vi "Measure.vi"(8 "error in (no error)":errorcluster, 11 "QPS settings":T1={"TWM pipe name"="\\\\.\\pipe\\TWM:server", "Measurement properties"={"Measurement ID"=enum."1", "Description"="3 phase, 3 ADC, 1 PJVS", "Switching matrix M"=[], "Signal frequency  (Hz)"=50.0, "Signal amplitudes (V)"=[], "PRs"=1, "PRe"=10, "MRs"=0, "MRe"=0, "Set PJVS frequency (Hz)"=50.0, "PJVS reference voltages (1 period, V)"=[], "Requiested PJVS steps"=10, "Sampling f (Hz)"=7000.0}, "PJVS setup"={"PJVS type"=enum."AC-supraVOLTcontrol", "Status Refnum"=refnum, "Abort Refnum"=refnum, "AC-supraVOLTcontrol"={"IP address:port (0.0.0.0:0000)"="0.0.0.0:0000", "Timeouts"={"TCP Read & Write (ms)"=7000, "Sensors readout"=5000, "PJVS setup"=10000, "Nullmeter readout"=5000, "Multiplexer setup"=3000, "57XX setup"=15000, "Generator setup"=5000, "Synthesizer setup"=3000, "Sampler readout"=10000}, "Simulation mode"=FALSE, "Debug mode"=FALSE}, "NPL bias source"={"Server name"="CZC", "Bias setup file"=path ""}}} {"Measurement properties"."PJVS reference voltages (1 period, V)" format="%.9g"}) -> (0 "error out":errorcluster, 3 "QPS settings out":T1={"TWM pipe name"="\\\\.\\pipe\\TWM:server", "Measurement properties"={"Measurement ID"=enum."1", "Description"="3 phase, 3 ADC, 1 PJVS", "Switching matrix M"=[], "Signal frequency  (Hz)"=50.0, "Signal amplitudes (V)"=[], "PRs"=1, "PRe"=10, "MRs"=0, "MRe"=0, "Set PJVS frequency (Hz)"=50.0, "PJVS reference voltages (1 period, V)"=[], "Requiested PJVS steps"=10, "Sampling f (Hz)"=7000.0}, "PJVS setup"={"PJVS type"=enum."AC-supraVOLTcontrol", "Status Refnum"=refnum, "Abort Refnum"=refnum, "AC-supraVOLTcontrol"={"IP address:port (0.0.0.0:0000)"="0.0.0.0:0000", "Timeouts"={"TCP Read & Write (ms)"=7000, "Sensors readout"=5000, "PJVS setup"=10000, "Nullmeter readout"=5000, "Multiplexer setup"=3000, "57XX setup"=15000, "Generator setup"=5000, "Synthesizer setup"=3000, "Sampler readout"=10000}, "Simulation mode"=FALSE, "Debug mode"=FALSE}, "NPL bias source"={"Server name"="CZC", "Bias setup file"=path ""}}} {"Measurement properties"."PJVS reference voltages (1 period, V)" format="%.9g"})   [LabVIEW 2020]
uses:
  external libraries/TWM client.lvlibp
  Type definitions/Measurement ID.ctl
  Type definitions/Measuement properties.ctl
  General PJVS driver/Type definitions/PJVS Type.ctl
  PJVS drivers/acsvcontrol-driver/build/ACSVcontrol-driver_0.2.0.0.llb/Timeouts.ctl
  PJVS drivers/acsvcontrol-driver/build/ACSVcontrol-driver_0.2.0.0.llb/ACSVcontrol-driver.lvlib
  General PJVS driver/Type definitions/PJVS Setup.ctl
  General PJVS driver/QPSsettings.ctl
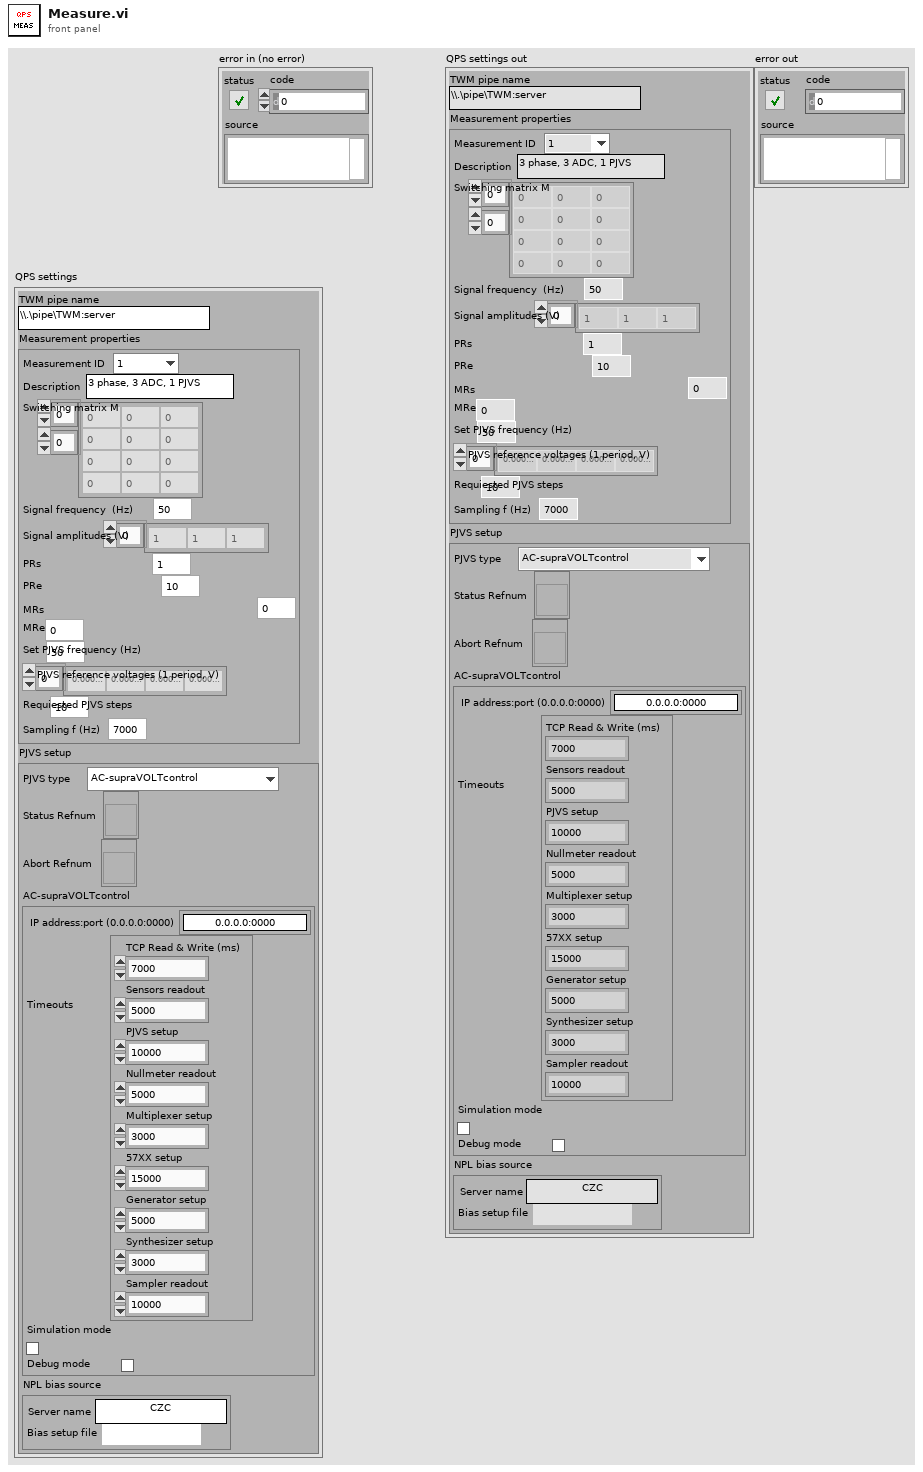
[diagram p1: front panel]
types:
  T1 = typedef "QPSsettings.ctl" = cluster{"TWM pipe name":string, "Measurement properties":T2, "PJVS setup":T4}
  T2 = typedef "Measuement properties.ctl" = cluster{"Measurement ID":T3, "Description":string, "Switching matrix M":i32[][], "Signal frequency  (Hz)":dbl, "Signal amplitudes (V)":dbl[], "PRs":i32, "PRe":i32, "MRs":i32, "MRe":i32, "Set PJVS frequency (Hz)":dbl, "PJVS reference voltages (1 period, V)":dbl[], "Requiested PJVS steps":i32, "Sampling f (Hz)":dbl}
  T3 = typedef "Measurement ID.ctl" = enum16{"M", "1", "2", "3"}
  T4 = typedef "PJVS Setup.ctl" = cluster{"PJVS type":T5, "Status Refnum":refnum<vi>, "Abort Refnum":refnum<vi>, "AC-supraVOLTcontrol":cluster{"IP address:port (0.0.0.0:0000)":string, "Timeouts":T6, "Simulation mode":bool, "Debug mode":bool}, "NPL bias source":cluster{"Server name":string, "Bias setup file":path}}
  T5 = typedef "PJVS Type.ctl" = enum16{"AC-supraVOLTcontrol", "NPL bias source"}
  T6 = typedef "ACSVcontrol-driver.lvlib/Timeouts.ctl" = cluster{"TCP Read & Write (ms)":i32, "Sensors readout":i32, "PJVS setup":i32, "Nullmeter readout":i32, "Multiplexer setup":i32, "57XX setup":i32, "Generator setup":i32, "Synthesizer setup":i32, "Sampler readout":i32}
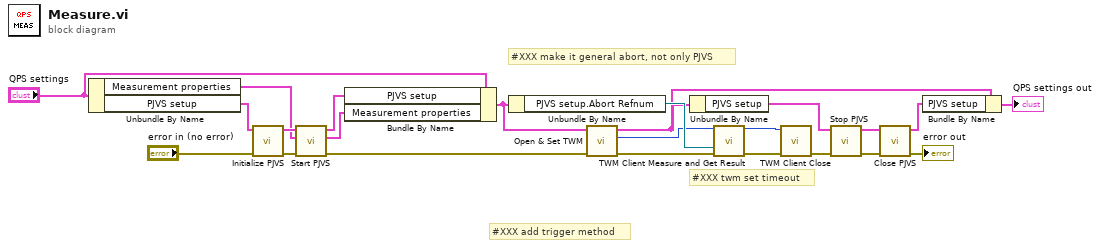
[diagram p0: block diagram]
diagram:
  # "#XXX add trigger method"
  # "#XXX twm set timeout"
  # "#XXX make it general abort, not only PJVS"
  n1 = Unbundle By Name("QPS settings") -> ("Measurement properties"=w18:T2, "PJVS setup"=w17:T4)
  n2 = call "Initialize PJVS.vi"("error in (no error)"="error in (no error)", "PJVS setup"=w17) -> ("error out"=w22:errorcluster, "PJVS setup out"=w23:T4)  [unwired: 8 in]
  n3 = call "Start PJVS.vi"("error in (pass through)"=w22, "Measurement properties"=w18, "PJVS setup"=w23) -> ("error out"=w12:errorcluster, "Measurement properties out"=w13:T2, "PJVS setup out"=w14:T4)  [unwired: 6 in]
  n4 = Bundle By Name(cluster="QPS settings", "PJVS setup"=w14, "Measurement properties"=w13) -> (w11:T1)
  n5 = Unbundle By Name(w11) -> ("PJVS setup.Abort Refnum"=w10:refnum<vi>)
  n6 = call "Open & Set TWM.vi"("error in"=w12, "QPS settings"=w11) -> ("error out"=w4:errorcluster, "TWM handle out"=w3:i32, "QPS settings out"=w7:T1)  [unwired: 7 in]
  n7 = Unbundle By Name(w7) -> ("PJVS setup"=w8:T4)
  n8 = call "TWM Client Measure and Get Result.vi"("handle"=w3, "stop ref (none)"=w10, "error in"=w4) -> ("handle out"=w1:i32, "error out"=w2:errorcluster)  [unwired: 8 in, 3 out]
  n9 = call "TWM Client Close.vi"("error in"=w2, "handle in"=w1) -> ("error out"=w9:errorcluster)  [unwired: 9 in]
  n10 = call "Stop PJVS.vi"("error in (pass through)"=w9, "PJVS setup"=w8) -> ("error out"=w21:errorcluster, "PJVS setup out"=w20:T4)  [unwired: 8 in]
  n11 = call "Close PJVS.vi"("error in (pass through)"=w21, "PJVS setup"=w20) -> ("error out"=→"error out":errorcluster, "PJVS setup out"=w6:T4)  [unwired: 8 in]
  n12 = Bundle By Name(cluster=w7, "PJVS setup"=w6) -> (→"QPS settings out":T1)
